vi "Lua.vi"(0 "Lua Version":enum16{"luajit", "jnlua"}(ring)=enum."jnlua", 1 "Action":enum16{"Open", "Load", "Start", "Run", "Close"}(ring), 2 "L In":u64, 3 "Name":string, 4 "Arg":variant) -> (5 "Lua Dll":path, 6 "L Out":u64, 7 "Status":string)   [LabVIEW 2014]
panel:
  in  "VIs":variant
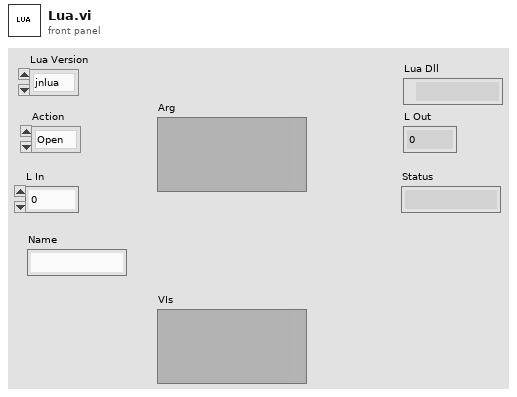
[diagram p1: front panel]
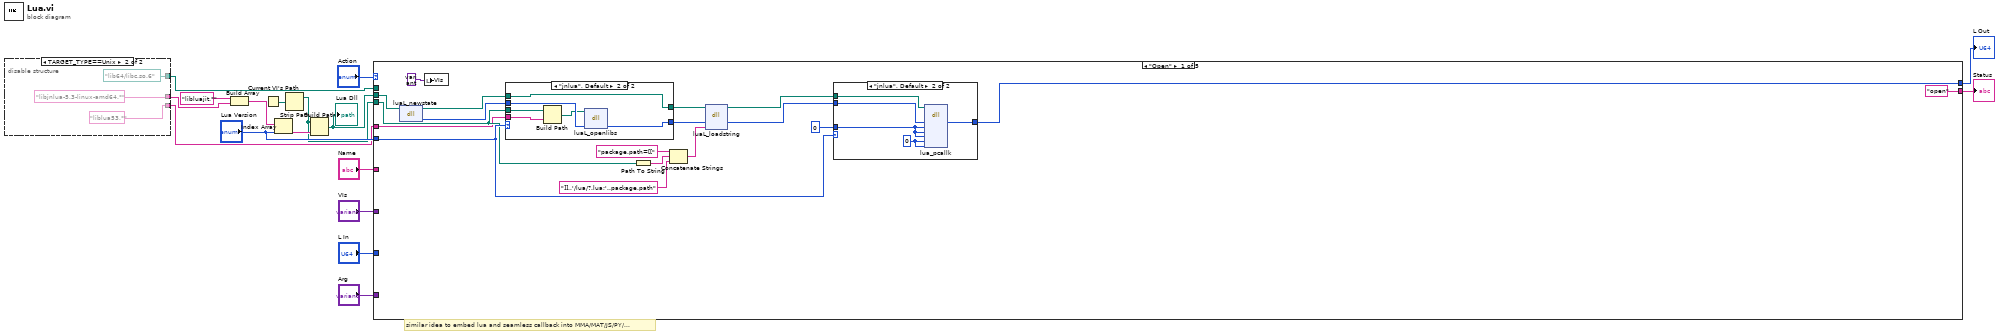
[diagram p0: block diagram]
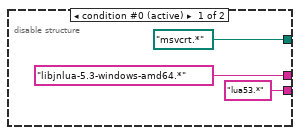
[diagram p2: hidden frame]
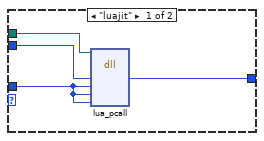
[diagram p3: hidden frame]
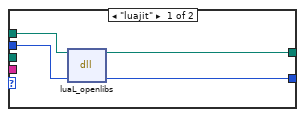
[diagram p4: hidden frame]
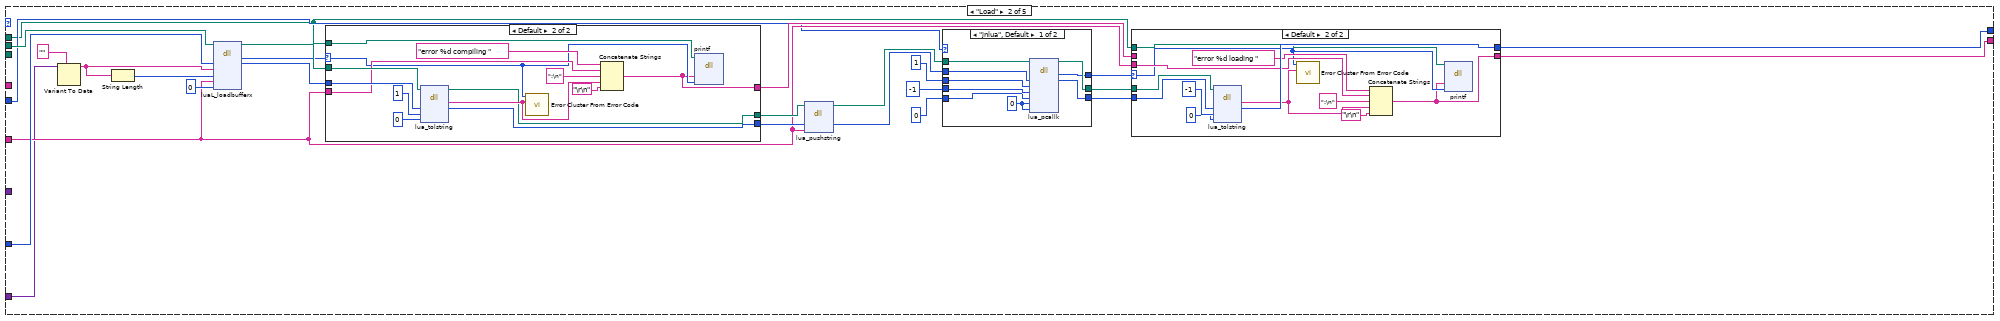
[diagram p5: hidden frame]
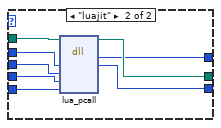
[diagram p6: hidden frame]
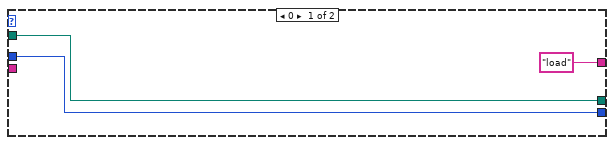
[diagram p7: hidden frame]
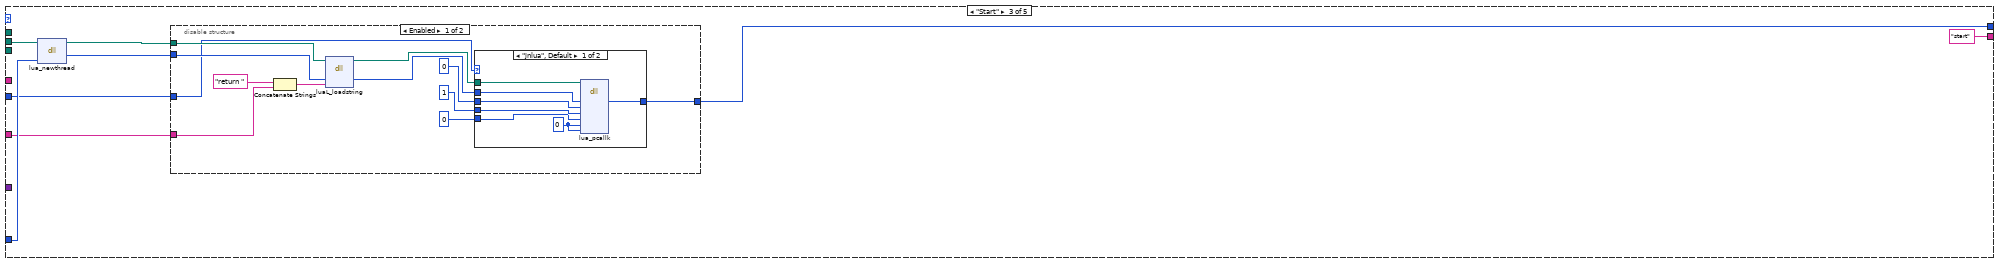
[diagram p9: hidden frame]
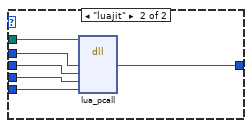
[diagram p10: hidden frame]
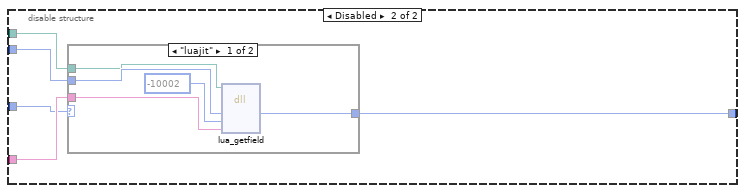
[diagram p11: hidden frame]
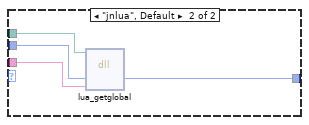
[diagram p12: hidden frame]
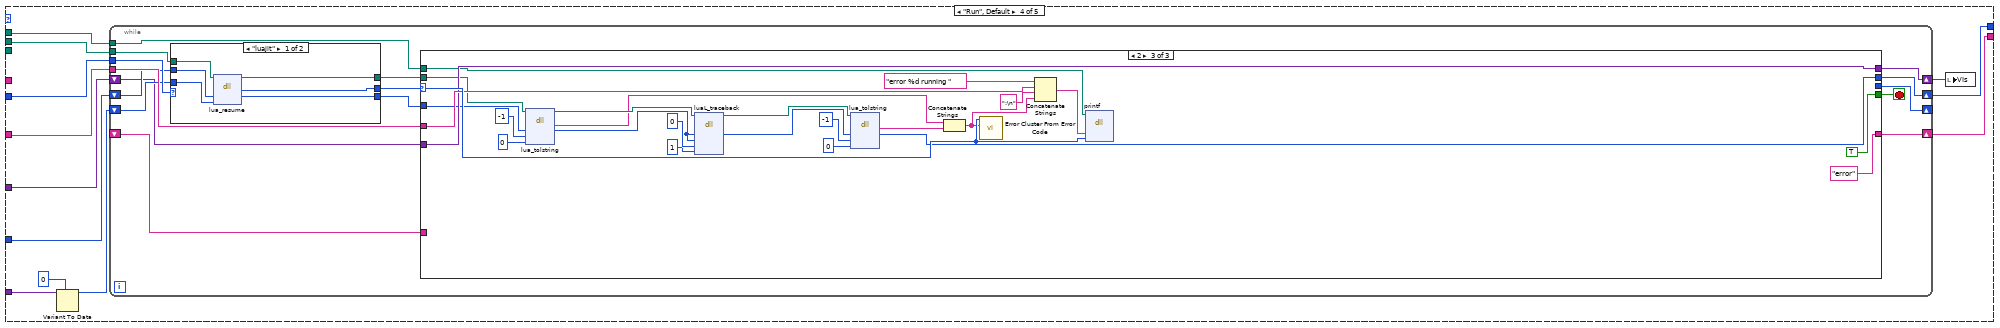
[diagram p13: hidden frame]
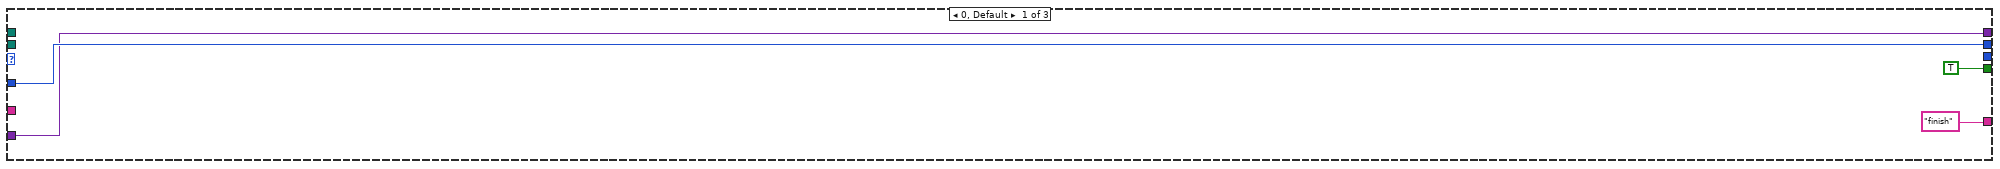
[diagram p14: hidden frame]
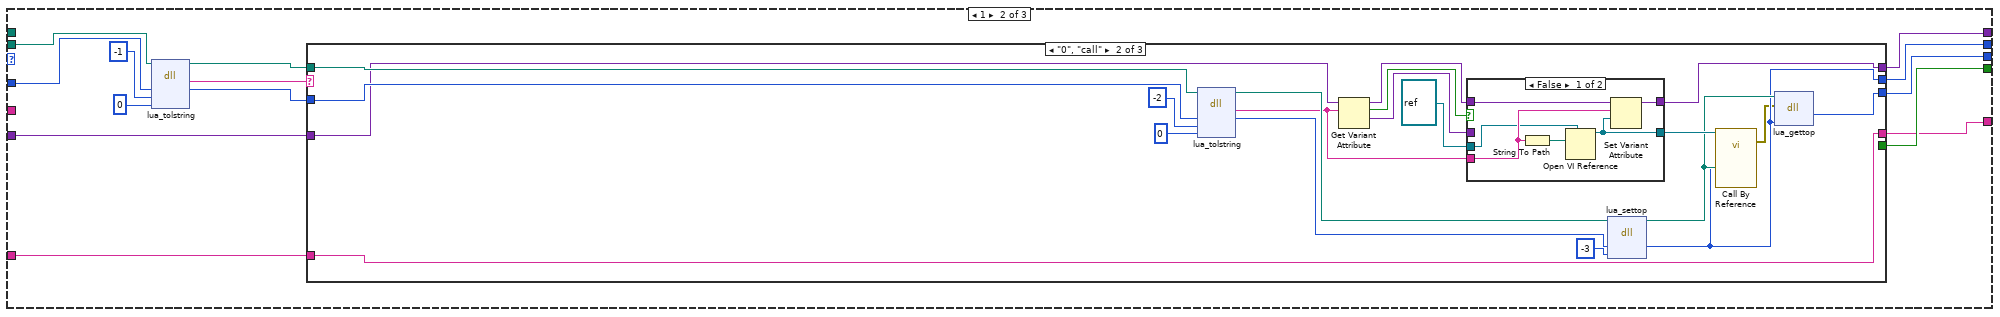
[diagram p15: hidden frame]
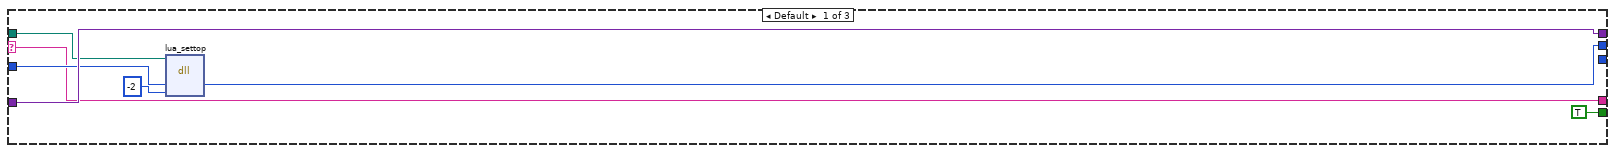
[diagram p16: hidden frame]
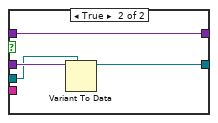
[diagram p17: hidden frame]
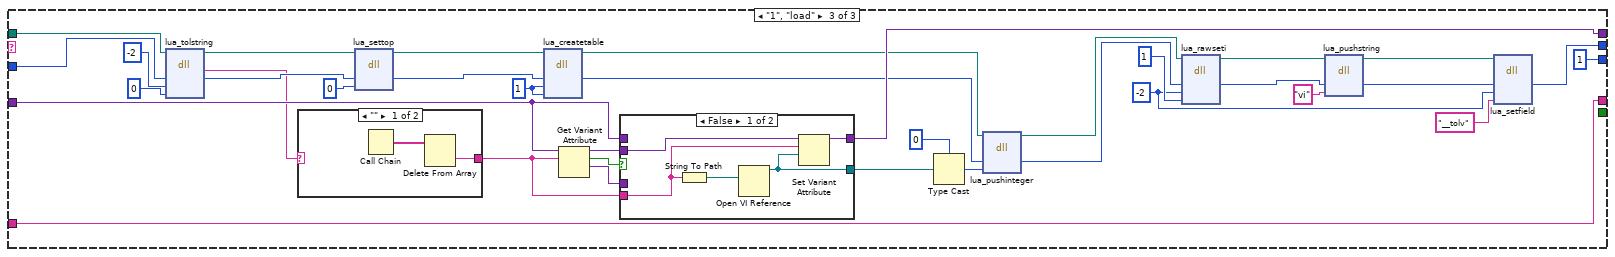
[diagram p18: hidden frame]
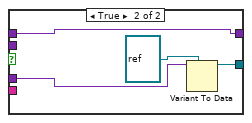
[diagram p20: hidden frame]
diagram:
  # "similar idea to embed lua and seamless callback into MMA/MAT/JS/PY/..."
  n1 = disable-structure shown="TARGET_TYPE==Unix" {
    disable-tunnel: ["libjnlua-5.3-windows-amd64.*" ("name or relative path") "libjnlua-5.3-linux-amd64.*" ("name or relative path")] -> w4
    disable-tunnel: ["lua53.*" ("name or relative path") "liblua53.*" ("name or relative path")] -> w2
    disable-tunnel: [path "msvcrt.*" ("path in") path "/lib64/libc.so.6" ("path in")] -> w1
    frame condition #0 (active) {
    }
    frame condition #1 {
    }
  }
  n2 = Build Array("libluajit.*" ("name or relative path"), w4) -> (w3:string[])
  n3 = Current VI's Path() -> (path=w16:path)
  n4 = Index Array(array=w3, index="Lua Version") -> (element=w15:string)
  n5 = Strip Path(path=w16) -> (stripped path=w6:path)  [unwired: 1 out]
  n6 = Build Path(base path=w6, name or relative path=w15) -> (appended path=w9:path)
  "Lua Dll" <- w9
  n7 = case shown="\"Open\"" "Action" {
    tunnel: [w31 w69 w139 w191 w354] -> w12
    tunnel: w9 -> [w32 w70 w142 w194 w355]
    tunnel: "L In" -> [_ w71 w141 w193 w356]
    tunnel: w6 -> [w25 _ _ _ _]
    tunnel: "Lua Version" -> [w28 w62 w140 w192 _]
    tunnel: "Name" -> [_ w68 w138 w190 _]
    tunnel: "Arg" -> [_ w67 _ w187 _]
    tunnel: "VIs" -> [_ _ _ w186 w353]
    tunnel: ["open" w64 "start" w184 "close"] -> w7
    tunnel: w1 -> [_ w61 _ w183 _]
    tunnel: w2 -> [w24 _ _ _ _]
    frame "Open" {
      n8 = dll-call lib="lua5.dll" fn="luaL_newstate"(path in=w32) -> (path out=w27:path, "L"=w33:u64)  [unwired: 2 in, 1 out]
      n9 = local write "VIs"(variant ("VIs")) -> ()
      n10 = case shown="\"jnlua\", Default" w28 {
        tunnel: [w53 w58] -> w36
        tunnel: [w51 w60] -> w35
        tunnel: w27 -> [w54 w58]
        tunnel: w33 -> [w52 w59]
        tunnel: w25 -> [_ w57]
        tunnel: w24 -> [_ w55]
        frame "luajit" {
          n11 = dll-call lib="lua5.dll" fn="luaL_openlibs"(path in=w54, "L"=w52) -> (path out=w53:path, "L"=w51:u64)  [unwired: 3 in, 1 out]
        }
        frame "jnlua", Default {
          n12 = Build Path(base path=w57, name or relative path=w55) -> (appended path=w56:path)
          n13 = dll-call lib="lua5.dll" fn="luaL_openlibs"(path in=w56, "L"=w59) -> ("L"=w60:u64)  [unwired: 3 in, 2 out]
        }
      }
      n14 = Path To String(path=w25) -> (string=w41:string)
      n15 = Concatenate Strings("package.path=[[" ("string"), w41, "]]..'/lua/?.lua;'..package.path" ("string")) -> (w40:string)
      n16 = dll-call lib="lua5.dll" fn="luaL_loadstring"(path in=w36, "L"=w35, "str"=w40) -> (path out=w37:path, "L"=w34:u64)  [unwired: 4 in, 1 out]
      n17 = case shown="\"jnlua\", Default" w28 {
        tunnel: w37 -> [w45 w46]
        tunnel: w34 -> [w43 w50]
        tunnel: [w44 w49] -> w31
        tunnel: 0 ("nresults") -> [w42 w47]
        frame "luajit" {
          n18 = dll-call lib="lua5.dll" fn="lua_pcall"(path in=w45, "L"=w43, "nargs"=w42, "nresults"=w42, "errfunc"=w42) -> ("L"=w44:u64)  [unwired: 6 in, 2 out]
        }
        frame "jnlua", Default {
          w48 = 0 ("nresults")
          n19 = dll-call lib="lua5.dll" fn="lua_pcallk"(path in=w46, "L"=w50, "nargs"=w47, "nresults"=w47, "errfunc"=w47, "arg5"=w48, "arg6"=w48) -> ("L"=w49:u64)  [unwired: 8 in, 2 out]
        }
      }
    }
    frame "Load" {
      n20 = Variant To Data(type="" ("string"), Variant=w67) -> (data=w65:string)  [unwired: 1 in, 1 out]
      n21 = String Length(string=w65) -> (length=w72:i32)
      n22 = dll-call lib="lua5.dll" fn="luaL_loadbufferx"(path in=w70, "L"=w71, "buff"=w65, "sz"=w72, "name"=w68, "mode"=u64 0) -> (path out=w77:path, "err"=w73:i32, "L"=w75:u64)  [unwired: 6 in, 1 out]
      n23 = case shown="Default" w73 {
        selector: w73 -> [_ w110]
        tunnel: w77 -> [w106 w116]
        tunnel: [w106 w109] -> w76
        tunnel: w75 -> [w105 w115]
        tunnel: [w105 w112] -> w74
        tunnel: w68 -> [_ w113]
        tunnel: ["load" w108] -> w63
        tunnel: w61 -> [_ w107]
        frame 0 {
        }
        frame Default {
          n24 = dll-call lib="lua5.dll" fn="lua_tolstring"(path in=w116, "L"=w115, "idx"=1, "len"=0) -> (path out=w109:path, "str"=w111:string, "L"=w112:u64)  [unwired: 4 in, 1 out]
          n25 = call <vilib>:"Error Cluster From Error Code.vi"("error message (\"\")"=w111, "error code (0)"=w110) -> ()  [unwired: 7 in, 1 out]
          n26 = Concatenate Strings("error %d compiling " ("string"), w113, ":\n" ("string"), w111, "\r\n") -> (w108:string)
          n27 = dll-call lib="lib64/libc.so.6" fn="printf"(path in=w107, "arg1"=w108, "arg2"=w110) -> ()  [unwired: 5 in, 2 out]
        }
      }
      n28 = dll-call lib="lua5.dll" fn="lua_pushstring"(path in=w76, "L"=w74, "str"=w68) -> (path out=w79:path, "L"=w78:u64)  [unwired: 4 in, 1 out]
      n29 = case shown="\"jnlua\", Default" w62 {
        tunnel: -1 ("nresults") -> [w95 w103]
        tunnel: 1 ("nresults") -> [w94 w102]
        tunnel: 0 ("errfunc") -> [w93 w101]
        tunnel: [w92 w100] -> w82
        tunnel: [w91 w99] -> w81
        tunnel: [w90 w98] -> w80
        tunnel: w79 -> [w88 w97]
        tunnel: w78 -> [w89 w96]
        frame "jnlua", Default {
          w87 = 0 ("errfunc")
          n30 = dll-call lib="lua5.dll" fn="lua_pcallk"(path in=w88, "L"=w89, "nargs"=w94, "nresults"=w95, "errfunc"=w93, "arg5"=w87, "arg6"=w87) -> (path out=w92:path, "err"=w90:i32, "L"=w91:u64)  [unwired: 7 in, 1 out]
        }
        frame "luajit" {
          n31 = dll-call lib="lua5.dll" fn="lua_pcall"(path in=w97, "L"=w96, "nargs"=w102, "nresults"=w103, "errfunc"=w101) -> (path out=w100:path, "err"=w98:i32, "L"=w99:u64)  [unwired: 5 in, 1 out]
        }
      }
      n32 = case shown="Default" w80 {
        selector: w80 -> [_ w125]
        tunnel: w82 -> [_ w130]
        tunnel: w81 -> [w122 w129]
        tunnel: [w122 w133] -> w69
        tunnel: w68 -> [_ w127]
        tunnel: [w121 w124] -> w64
        tunnel: w63 -> [w121 _]
        tunnel: w61 -> [_ w123]
        frame 0 {
        }
        frame Default {
          n33 = dll-call lib="lua5.dll" fn="lua_tolstring"(path in=w130, "L"=w129, "idx"=-1, "len"=0) -> ("str"=w126:string, "L"=w133:u64)  [unwired: 4 in, 2 out]
          n34 = call <vilib>:"Error Cluster From Error Code.vi"("error message (\"\")"=w126, "error code (0)"=w125) -> ()  [unwired: 7 in, 1 out]
          n35 = Concatenate Strings("error %d loading " ("string"), w127, ":\n" ("string"), w126, "\r\n") -> (w124:string)
          n36 = dll-call lib="lib64/libc.so.6" fn="printf"(path in=w123, "arg1"=w124, "arg2"=w125) -> ()  [unwired: 5 in, 2 out]
        }
      }
    }
    frame "Start" {
      n37 = dll-call lib="lua5.dll" fn="lua_newthread"(path in=w142, "L"=w141) -> (path out=w143:path, "thread"=w137:u64)  [unwired: 3 in, 1 out]
      n38 = disable-structure shown="Enabled" {
        disable-tunnel: w137 -> [w155 w171]
        disable-tunnel: w143 -> [w154 w173]
        disable-tunnel: [w151 w172] -> w139
        disable-tunnel: w138 -> [w148 w170]
        disable-tunnel: w140 -> [w147 w169]
        frame Enabled {
          n39 = Concatenate Strings("return " ("str"), w148) -> (w149:string)
          n40 = dll-call lib="lua5.dll" fn="luaL_loadstring"(path in=w154, "L"=w155, "str"=w149) -> (path out=w153:path, "L"=w152:u64)  [unwired: 4 in, 1 out]
          n41 = case shown="\"jnlua\", Default" w147 {
            tunnel: w153 -> [w156 w168]
            tunnel: w152 -> [w162 w167]
            tunnel: [w161 w166] -> w151
            tunnel: 0 ("nargs") -> [w160 w165]
            tunnel: 1 ("nresults") -> [w159 w164]
            tunnel: 0 ("errfunc") -> [w158 w163]
            frame "jnlua", Default {
              w157 = 0 ("errfunc")
              n42 = dll-call lib="lua5.dll" fn="lua_pcallk"(path in=w156, "L"=w162, "nargs"=w160, "nresults"=w159, "errfunc"=w158, "arg5"=w157, "arg6"=w157) -> ("L"=w161:u64)  [unwired: 8 in, 2 out]
            }
            frame "luajit" {
              n43 = dll-call lib="lua5.dll" fn="lua_pcall"(path in=w168, "L"=w167, "nargs"=w165, "nresults"=w164, "errfunc"=w163) -> ("L"=w166:u64)  [unwired: 6 in, 2 out]
            }
          }
        }
        frame Disabled {
          n44 = case shown="\"luajit\"" w169 {
            tunnel: w171 -> [w177 w182]
            tunnel: w173 -> [w176 w181]
            tunnel: [w175 w180] -> w172
            tunnel: w170 -> [w178 w179]
            frame "luajit" {
              n45 = dll-call lib="lua5.dll" fn="lua_getfield"(path in=w176, "L"=w177, "idx"=-10002, "name"=w178) -> ("L"=w175:u64)  [unwired: 5 in, 2 out]
            }
            frame "jnlua", Default {
              n46 = dll-call lib="lua5.dll" fn="lua_getglobal"(path in=w181, "L"=w182, "name"=w179) -> ("L"=w180:u64)  [unwired: 4 in, 2 out]
            }
          }
        }
      }
    }
    frame "Run", Default {
      n47 = Variant To Data(type=0 ("int"), Variant=w187) -> (data=w189:i32)  [unwired: 1 in, 1 out]
      n48 = while {
        tunnel: w194 -> [w203]
        tunnel: w192 -> [w208]
        shift-right: [w207] -> w191
        shift-left: w193 -> [w202]
        tunnel: w190 -> [w204]
        shift-right: [w200] -> _
        shift-left: w189 -> [w201]
        shift-right: [w199] -> w185
        shift-left: w186 -> [w198]
        shift-right: [w197] -> w184
        shift-left: _ -> [w196]
        tunnel: w183 -> [w195]
        stop <- w205 stop-if-true
        n49 = case shown="\"luajit\"" w208 {
          tunnel: w203 -> [w343 w346]
          tunnel: w202 -> [w340 w345]
          tunnel: [w341 w350] -> w209
          tunnel: [w342 w349] -> w206
          tunnel: [w339 w347] -> w210
          tunnel: w201 -> [w338 w344]
          frame "luajit" {
            n50 = dll-call lib="lua5.dll" fn="lua_resume"(path in=w343, "L"=w340, "narg"=w338) -> (path out=w339:path, "err"=w342:i32, "L"=w341:u64)  [unwired: 3 in, 1 out]
          }
          frame "jnlua", Default {
            n51 = dll-call lib="lua5.dll" fn="lua_resume"(path in=w346, "L"=w345, "from"=u64 0, "narg"=w344) -> (path out=w347:path, "err"=w349:i32, "L"=w350:u64)  [unwired: 4 in, 1 out]
          }
        }
        n52 = case shown="2" w206 {
          selector: w206 -> [_ _ w330]
          tunnel: w210 -> [_ w223 w324]
          tunnel: w209 -> [w213 w221 w322]
          tunnel: [w213 w228 w328] -> w207
          tunnel: [TRUE w227 TRUE] -> w205
          tunnel: w204 -> [_ _ w327]
          tunnel: [_ w226 _] -> w200
          tunnel: [w212 w225 w326] -> w199
          tunnel: w198 -> [w212 w224 w326]
          tunnel: ["finish" w216 "error"] -> w197
          tunnel: w196 -> [_ w215 _]
          tunnel: w195 -> [_ _ w313]
          frame 0, Default {
          }
          frame 1 {
            n53 = dll-call lib="lua5.dll" fn="lua_tolstring"(path in=w223, "L"=w221, "idx"=-1, "len"=0) -> (path out=w222:path, "str"=w217:string, "L"=w220:u64)  [unwired: 4 in, 1 out]
            n54 = case shown="\"0\", \"call\"" w217 {
              selector: w217 -> [w229 _ _]
              tunnel: [w231 w237 w274] -> w228
              tunnel: w224 -> [w234 w248 w292]
              tunnel: [w234 w241 w291] -> w225
              tunnel: w222 -> [w233 w253 w290]
              tunnel: w220 -> [w232 w250 w289]
              tunnel: [TRUE _ _] -> w227
              tunnel: [w229 w240 w269] -> w216
              tunnel: w215 -> [_ w240 w269]
              tunnel: [_ w239 1] -> w226
              frame Default {
                n55 = dll-call lib="lua5.dll" fn="lua_settop"(path in=w233, "L"=w232, "idx"=-2) -> ("L"=w231:u64)  [unwired: 4 in, 2 out]
              }
              frame "0", "call" {
                n56 = dll-call lib="lua5.dll" fn="lua_tolstring"(path in=w253, "L"=w250, "idx"=-2, "len"=0) -> (path out=w252:path, "str"=w245:string, "L"=w249:u64)  [unwired: 4 in, 1 out]
                n57 = Get Variant Attribute(Variant=w248, name=w245) -> (duplicate Variant=w244:variant, found=w247:bool, value=w246:variant)  [unwired: 2 in, 1 out]
                n58 = case shown="False" w247 {
                  tunnel: w245 -> [w261 _]
                  tunnel: w246 -> [_ w265]
                  tunnel: w244 -> [w258 w264]
                  tunnel: [w256 w262] -> w242
                  tunnel: refnum<vi> refnum ("type specifier VI Refnum (for type only)") -> [w259 w263]
                  tunnel: [w257 w264] -> w241
                  frame False {
                    n59 = String To Path(string=w261) -> (path=w260:path)
                    n60 = Open VI Reference(type specifier VI Refnum (for type only)=w259, vi path=w260) -> (vi reference=w256:refnum<vi>)  [unwired: 4 in, 1 out]
                    n61 = Set Variant Attribute(Variant=w258, name=w261, value=w256) -> (Variant out=w257:variant)  [unwired: 1 in, 2 out]
                  }
                  frame True {
                    n62 = Variant To Data(type=w263, Variant=w265) -> (data=w262:refnum<vi>)  [unwired: 1 in, 1 out]
                  }
                }
                n63 = dll-call lib="lua5.dll" fn="lua_settop"(path in=w252, "L"=w249, "idx"=-3) -> (path out=w238:path, "L"=w237:u64)  [unwired: 4 in, 1 out]
                n64 = call-by-ref "?"(reference=w242, "L"=w237, "Path"=w238) -> (error out=w236:errorcluster)  [unwired: 1 in, 1 out]
                n65 = dll-call lib="lua5.dll" fn="lua_gettop"(path in=w238, error in=w236, "L"=w237) -> (w239:i32)  [unwired: 2 in, 2 out]
              }
              frame "1", "load" {
                w277 = 1 ("narr")
                w280 = -2 ("n")
                n66 = dll-call lib="lua5.dll" fn="lua_tolstring"(path in=w290, "L"=w289, "idx"=-2, "len"=0) -> (path out=w294:path, "str"=w267:string, "L"=w293:u64)  [unwired: 4 in, 1 out]
                n67 = case shown="\"\"" w267 {
                  selector: w267 -> [_ w303]
                  tunnel: [w301 w303] -> w266
                  frame "" {
                    n68 = Call Chain() -> (call chain=w302:string[])
                    n69 = Delete From Array(array=w302) -> (deleted portion=w301:string)  [unwired: 2 in, 1 out]
                  }
                  frame Default {
                  }
                }
                n70 = dll-call lib="lua5.dll" fn="lua_settop"(path in=w294, "L"=w293, "idx"=0) -> (path out=w276:path, "L"=w275:u64)  [unwired: 4 in, 1 out]
                n71 = dll-call lib="lua5.dll" fn="lua_createtable"(path in=w276, "L"=w275, "narr"=w277, "nrec"=w277) -> (path out=w279:path, "L"=w278:u64)  [unwired: 5 in, 1 out]
                n72 = Get Variant Attribute(Variant=w292, name=w266) -> (duplicate Variant=w295:variant, found=w297:bool, value=w296:variant)  [unwired: 2 in, 1 out]
                n73 = case shown="False" w297 {
                  tunnel: w292 -> [_ w311]
                  tunnel: w266 -> [w304 _]
                  tunnel: w296 -> [_ w312]
                  tunnel: w295 -> [w307 _]
                  tunnel: [w305 w309] -> w272
                  tunnel: [w306 w311] -> w291
                  frame False {
                    n74 = String To Path(string=w304) -> (path=w308:path)
                    n75 = Open VI Reference(vi path=w308) -> (vi reference=w305:refnum<vi>)  [unwired: 5 in, 1 out]
                    n76 = Set Variant Attribute(Variant=w307, name=w304, value=w305) -> (Variant out=w306:variant)  [unwired: 1 in, 2 out]
                  }
                  frame True {
                    n77 = Variant To Data(type=refnum<vi> refnum ("vi reference"), Variant=w312) -> (data=w309:refnum<vi>)  [unwired: 1 in, 1 out]
                  }
                }
                n78 = Type Cast(type=u32 0 ("i"), x=w272) -> (*(type *) &x=w271:u32)
                n79 = dll-call lib="lua5.dll" fn="lua_pushinteger"(path in=w279, "L"=w278, "n"=w271) -> (path out=w285:path, "L"=w283:u64)  [unwired: 4 in, 1 out]
                n80 = dll-call lib="lua5.dll" fn="lua_rawseti"(path in=w285, "L"=w283, "n"=w280, "i"=1) -> (path out=w284:path, "L"=w282:u64)  [unwired: 5 in, 1 out]
                n81 = dll-call lib="lua5.dll" fn="lua_pushstring"(path in=w284, "L"=w282, "str"="vi") -> (path out=w288:path, "L"=w287:u64)  [unwired: 4 in, 1 out]
                n82 = dll-call lib="lua5.dll" fn="lua_setfield"(path in=w288, "L"=w287, "n"=w280, "i"="__tolv") -> ("L"=w274:u64)  [unwired: 5 in, 2 out]
              }
            }
          }
          frame 2 {
            n83 = dll-call lib="lua5.dll" fn="lua_tolstring"(path in=w324, "L"=w322, "idx"=-1, "len"=0) -> (path out=w323:path, "str"=w317:string, "L"=w321:u64)  [unwired: 4 in, 1 out]
            n84 = dll-call lib="lua5.dll" fn="luaL_traceback"(path in=w323, "L"=w321, "L1"=w321, "msg"=0 ("level"), "level"=1) -> (path out=w334:path, "L"=w333:u64)  [unwired: 6 in, 1 out]
            n85 = dll-call lib="lua5.dll" fn="lua_tolstring"(path in=w334, "L"=w333, "idx"=-1, "len"=0) -> ("str"=w316:string, "L"=w328:u64)  [unwired: 4 in, 2 out]
            n86 = Concatenate Strings(w317, w316) -> (w315:string)
            n87 = call <vilib>:"Error Cluster From Error Code.vi"("error message (\"\")"=w315, "error code (0)"=w330) -> ()  [unwired: 7 in, 1 out]
            n88 = Concatenate Strings("error %d running " ("string"), w327, ":\n" ("string"), w315) -> (w318:string)
            n89 = dll-call lib="lib64/libc.so.6" fn="printf"(path in=w313, "arg1"=w318, "arg2"=w330) -> ()  [unwired: 5 in, 2 out]
          }
        }
      }
      n90 = local write "VIs"(w185) -> ()
    }
    frame "Close" {
      n91 = dll-call lib="lua5.dll" fn="lua_close"(path in=w355, "L"=w356) -> ("L"=w354:u64)  [unwired: 3 in, 2 out]
      n92 = Get Variant Attribute(Variant=w353) -> (values=w352:variant[])  [unwired: 3 in, 3 out]
      n93 = for {
        tunnel: w352 -> [w358] mode=indexing
        n94 = Variant To Data(type=refnum<vi> refnum ("vi reference"), Variant=w358) -> (data=w357:refnum<vi>)  [unwired: 1 in, 1 out]
        n95 = Close Reference(reference=w357) -> ()  [unwired: 1 in, 1 out]
      }
    }
  }
  "L Out" <- w12
  "Status" <- w7
